vi "Module ID.vi"(11 "Remote Messaging Module in":refnum<class "Remote Messaging Module.lvclass">) -> (2 "Module ID":string)   [LabVIEW 2020, in "Volatus.lvlib" / "Remote Messaging Module.lvclass"]
uses:
  Remote Messaging Module.lvclass
  Remote Messaging Module.lvclass/Remote Messaging Module.ctl
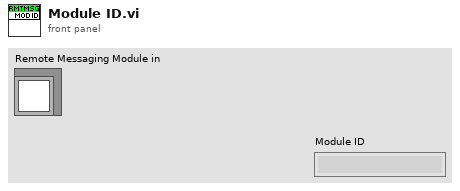
[diagram p1: front panel]
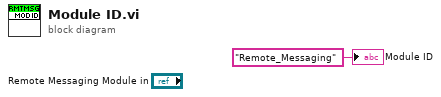
[diagram p0: block diagram]
diagram:
  "Module ID" <- "Remote_Messaging" ("Module ID")
